vi "Get ILC Data.vi"(11 "Model in":refnum<class "Model.lvclass">) -> (2 "ILCData":T1[](array[typedef]) {"Axial Pull Pressure" format="%.4f"; "Axial Push Pressure" format="%.4f"; "Lateral Pull Pressure" format="%.4f"; "Lateral Push Pressure" format="%.4f"; "Timestamp" format="%.4f"; "Lateral Force" format="%.4f"; "Axial Force" format="%.4f"; "FC2 Force" format="%.4f"; "FC1 Force" format="%.4f"}, 3 "Model out":refnum<class "Model.lvclass">)   [LabVIEW 2015, in "Model.lvclass"]
uses:
  Model.lvclass
  Typedefs/ActuatorData.ctl
  Model.lvclass/Model.ctl
  Typedefs/FAMT Typedefs.lvlib
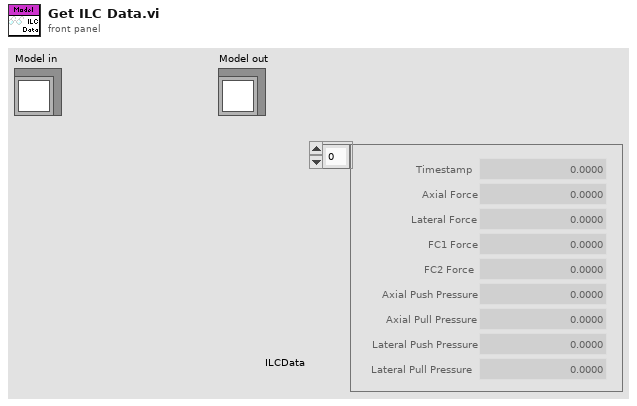
[diagram p1: front panel]
types:
  T1 = typedef "FAMT Typedefs.lvlib/ActuatorData.ctl" = cluster{"Timestamp":dbl, "Axial Force":dbl, "Lateral Force":dbl, "FC1 Force":dbl, "FC2 Force":dbl, "Lateral Push Pressure":dbl, "Lateral Pull Pressure":dbl, "Axial Push Pressure":dbl, "Axial Pull Pressure":dbl}
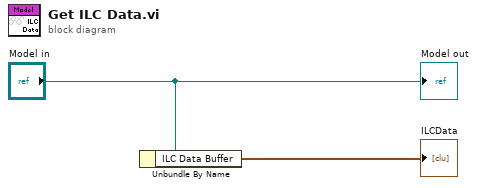
[diagram p0: block diagram]
diagram:
  n1 = Unbundle By Name("Model in") -> ("ILC Data Buffer"=→"ILCData":T1[])
  "Model out" <- "Model in"
